vi "get inventory from robot.vi"(8 "error in (no error)":errorcluster, 10 "Device selection":refnum<vi>) -> (0 "error out":errorcluster, 3 "Inventory":T1)   [LabVIEW 2016]
uses:
  Communication Global variables.vi
  <vilib>/addons/_JKI.lib/REST Client/classes/REST Client/REST Client.lvclass
  <vilib>/addons/_JKI.lib/Serialization/JSON/JKI JSON Serialization.lvlib
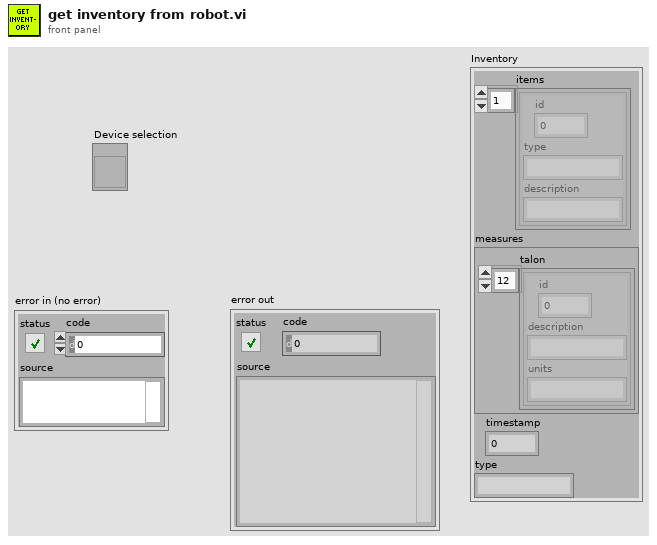
[diagram p1: front panel]
types:
  T1 = cluster{"items":cluster{"id":u8, "type":string, "description":string}[], "measures":cluster{"talon":cluster{"id":u8, "description":string, "units":string}[]}, "timestamp":i64, "type":string}
  T2 = cluster{"id":u8, "type":string, "description":string}[]
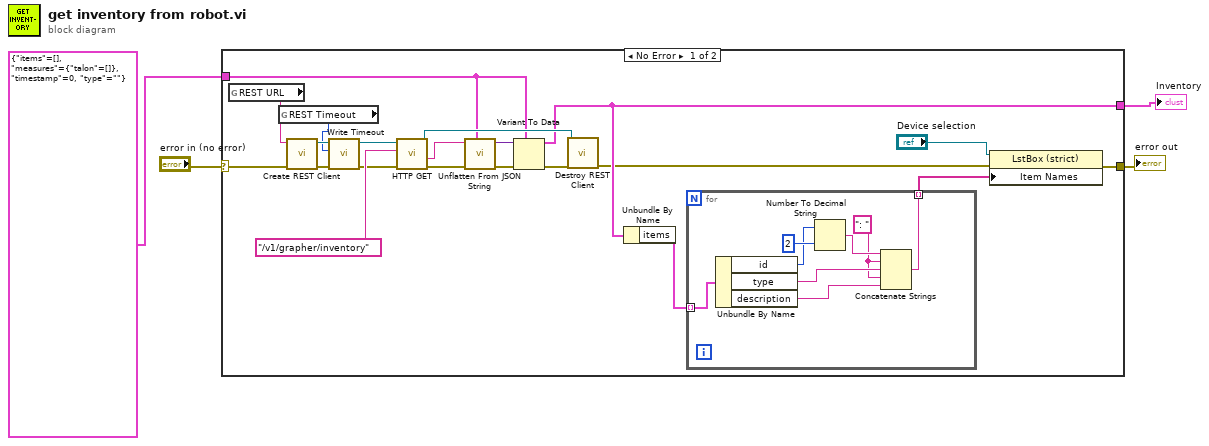
[diagram p0: block diagram]
diagram:
  n1 = case shown="No Error" "error in (no error)" {
    selector: "error in (no error)" -> [w25 w35]
    tunnel: [w18 w35] -> w3
    tunnel: T1 {"items"=[], "measures"={"talon"=[]}, "timestamp"=0, "type"=""} -> [w16 w34]
    tunnel: [w21 w34] -> w1
    frame No Error {
      n2 = global read "Communication Global variables.vi" "REST URL"() -> (w12:string)
      n3 = global read "Communication Global variables.vi" "REST Timeout"() -> (w5:i32)
      n4 = call <vilib>:"Create REST Client.vi"("error in (no error)"=w25, "Base URL"=w12) -> ("error out"=w9:errorcluster, "REST Client out"=w6:refnum<class "REST Client.lvclass">)  [unwired: 8 in]
      n5 = call-dynamic "Write Timeout.vi"("error in (no error)"=w9, "Timeout"=w5, "REST Client in"=w6) -> ("error out"=w8:errorcluster, "REST Client out"=w7:refnum<class "REST Client.lvclass">)  [unwired: 7 in]
      n6 = call-dynamic "HTTP GET.vi"("error in (no error)"=w8, "Path"="/v1/grapher/inventory", "REST Client in"=w7) -> ("error out"=w15:errorcluster, "Response body"=w13:string, "REST Client out"=w23:refnum<class "REST Client.lvclass">)  [unwired: 3 in, 3 out]
      n7 = call <vilib>:"Unflatten From JSON String.vi"("Type and Defaults"=w16, "error in (no error)"=w15, "JSON String"=w13) -> ("error out"=w14:errorcluster, "Variant"=w17:variant)  [unwired: 7 in]
      n8 = Variant To Data(error in=w14, type=w16, Variant=w17) -> (data=w21:T1, error out=w22:errorcluster)
      n9 = call-dynamic "Destroy REST Client.vi"("error in (no error)"=w22, "REST Client in"=w23) -> ("error out"=w19:errorcluster)  [unwired: 9 in]
      n10 = Unbundle By Name(w21) -> ("items"=w20:T2)
      n11 = for {
        tunnel: w20 -> [w33] mode=indexing
        tunnel: [w29] -> w10 mode=indexing
        w26 = ": " ("string")
        n12 = Unbundle By Name(w33) -> ("id"=w28:u8, "type"=w31:string, "description"=w32:string)
        n13 = Number To Decimal String(number=w28, width (-)=i16 2) -> (decimal integer string=w27:string)
        n14 = Concatenate Strings(w27, w26, w31, w26, w32) -> (w29:string)
      }
      n15 = property class="LstBox (strict)"(reference="Device selection", error in=w19, "Item Names"=w10) -> (error out=w18:errorcluster)  [unwired: 1 out]
    }
    frame Error {
    }
  }
  "error out" <- w3
  "Inventory" <- w1
